vi "AlliGator Python Plugin Valid Output Destination.vi"(2 "Output Destination":string) -> (7 "Valid Destination?":bool)   [LabVIEW 2021, in "AlliGator Python Plugins.lvlib"]
doc: "Checks whether the output destination is valid."
uses:
  AlliGator Python Plugins.lvlib
  Strings/Strings.lvlib
panel:
  # "see the AlliGator License on the block diagram (Ctrl+E or Window:Show Block Diagram)"
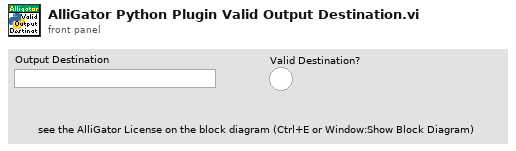
[diagram p1: front panel]
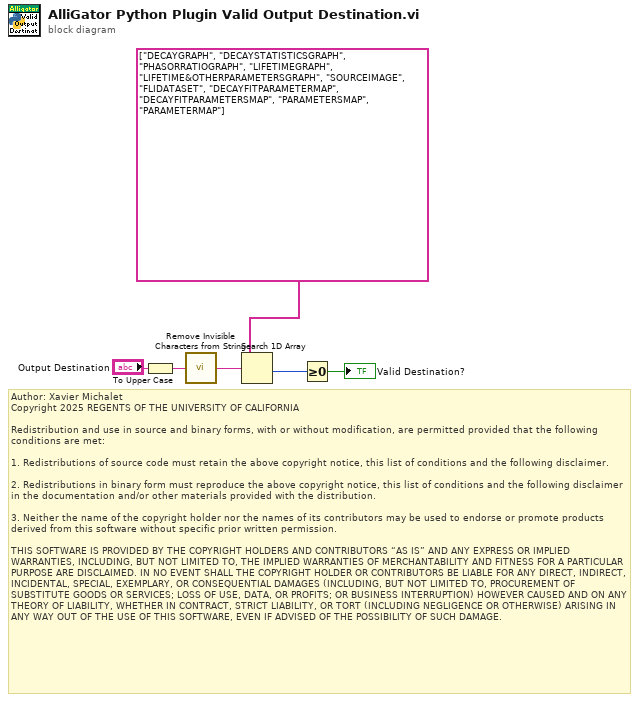
[diagram p0: block diagram]
diagram:
  # "Author: Xavier Michalet\nCopyright 2025 REGENTS OF THE UNIVERSITY OF CALIFORNIA\n\nRedistribution and use in source and binary forms, with or without modification, are permitted provided that the following conditions are met:\n\n1. Redistributions of source code must retain the above copyright notice, this list of conditions and the following disclaimer.\n\n2. Redistributions in binary form must reproduce the above copyright notice, this list of conditions and the following disclaimer in the documentation and/or other materials provided with the distribution.\n\n3. Neither the name of the copyright holder nor the names of its contributors may be used to endorse or promote products derived from this software without specific prior written permission.\n\nTHIS SOFTWARE IS PROVIDED BY THE COPYRIGHT HOLDERS AND CONTRIBUTORS “AS IS” AND ANY EXPRESS OR IMPLIED WARRANTIES, INCLUDING, BUT NOT LIMITED TO, THE IMPLIED WARRANTIES OF MERCHANTABILITY AND FITNESS FOR A PARTICULAR PURPOSE ARE DISCLAIMED. IN NO EVENT SHALL THE COPYRIGHT HOLDER OR CONTRIBUTORS BE LIABLE FOR ANY DIRECT, INDIRECT, INCIDENTAL, SPECIAL, EXEMPLARY, OR CONSEQUENTIAL DAMAGES (INCLUDING, BUT NOT LIMITED TO, PROCUREMENT OF SUBSTITUTE GOODS OR SERVICES; LOSS OF USE, DATA, OR PROFITS; OR BUSINESS INTERRUPTION) HOWEVER CAUSED AND ON ANY THEORY OF LIABILITY, WHETHER IN CONTRACT, STRICT LIABILITY, OR TORT (INCLUDING NEGLIGENCE OR OTHERWISE) ARISING IN ANY WAY OUT OF THE USE OF THIS SOFTWARE, EVEN IF ADVISED OF THE POSSIBILITY OF SUCH DAMAGE."
  n1 = To Upper Case(1:"Output Destination") -> (0:w4:string)
  n2 = call "Remove Invisible Characters from String.vi"("String"=w4) -> ("result string"=w1:string)  [unwired: 3 in]
  n3 = Search 1D Array(1D array=string[] ["DECAYGRAPH", "DECAYSTATISTICSGRAPH", "PHASORRATIOGRAPH", "LIFETIMEGRAPH", "LIFETIME&OTHERPARAMETERSGRAPH", "SOURCEIMAGE", "FLIDATASET", "DECAYFITPARAMETERMAP", "DECAYFITPARAMETERSMAP", "PARAMETERSMAP", "PARAMETERMAP"], element=w1) -> (index of element=w3:i32)  [unwired: 1 in]
  n4 = Greater Or Equal To 0?(x=w3) -> (x >= 0?=→"Valid Destination?":bool)
